vi "Dashboard Main.vi"() -> ()   [LabVIEW 2014]
uses:
  <vilib>/event_ctls.llb/eventvkey.ctl
  <vilib>/Utility/config.llb/NI_LVConfig.lvlib
  <vilib>/Utility/config.llb/Write Key (I32).vi
  <vilib>/Rock Robotics/WPI/Dashboard/WPI_DashboardLogging Global.vi
  <vilib>/Utility/config.llb/Write Key (String).vi
  <vilib>/Rock Robotics/Network Tables/SD Read Boolean.vi
  Support Files/Global Data!!!.vi
panel:
  in  "TCP":refnum<k5>
  in  "Rec Mode":enum32{"Stop", "Record", "Playback"}(radio)
  in  "Vision":u16(ring) items=["Camera Off", "USB Camera SW", "USB Camera HW", "IP Camera"]
  out "Camera IP":string
  out "Image Message":string="Timeout in Camera Communications"
  in  "Dashboard Tab":T1(tab)
  in  "Camera Settings":T2={"Frame Rate"=30, "Compression"=30, "Size"=1} {"Frame Rate" scale=1.0..30.0; "Size" items=["640x480", "320x240", "160x120"]}
  out "MotorChart R":cluster{"Numeric":dbl, "Numeric":dbl}(graph)
  out "MotorChart L":T3(graph)
  out "MotorSliders R":cluster{"MotorSlide1":dbl, "MotorSlide2":dbl} {"MotorSlide2" scale=-1.0..1.0 scale format="%#_2e"; "MotorSlide1" scale=-1.0..1.0 scale format="%#_2e"}
  out "MotorSliders L":T4 {"MotorSlide4 2" scale=0.0..14.0 scale format="%#_2e"; "MotorSlide2" scale=-1.0..1.0 scale format="%#_2e"; "MotorSlide1" scale=-1.0..1.0 scale format="%#_2e"}
  out "JS1 Z":dbl(slide) scale=-1.0..1.0 scale format="%#_2e"
  out "JS1 Graph":cluster{"X":dbl, "Y":dbl}[](graph)
  out "JS1 Buttons":T5
  out "JS2 Z":dbl(slide) scale=-1.0..1.0 scale format="%#_2e"
  out "JS2 Graph":cluster{"X":dbl, "Y":dbl}[](graph)
  out "JS2 Buttons":T5
  out "Mode":T6(ring)=enum."Auto Disabled"
  in  "DB Camera Config":bool
  out "fps":dbl format="%#.1g"
  out "Mbps":dbl format="%#.1g"
  out "Mbps 2":bool
  in  "DB/String 9":string
  in  "DB/String 8":string
  in  "DB/String 7":string
  in  "DB/String 6":string
  in  "DB/String 5":string
  in  "DB/String 4":string
  in  "DB/String 3":string
  in  "DB/String 2":string
  in  "DB/String 1":string
  in  "DB/String 0":string
  in  "DB/Slider 0":dbl(slide) scale=0.0..5.0
  in  "DB/Slider 1":dbl(slide) scale=0.0..5.0
  in  "DB/Slider 2":dbl(slide) scale=0.0..5.0
  in  "DB/Slider 3":dbl(slide) scale=0.0..5.0
  out "DB/LED 3":bool
  out "DB/LED 2":bool
  out "DB/LED 1":bool
  out "DB/LED 0":bool
  in  "DB/Button 3":bool
  in  "DB/Button 2":bool
  in  "DB/Button 1":bool
  in  "DB/Button 0":bool caption="New Name"
  out "BinTote":bool
  in  "Test Slider":dbl(slide) scale=0.0..100.0 scale format="%#_3g"
  in  "On/Off":bool caption="Solenoid"
  in  "Test Name":u16(ring) items=["Select the test to run...", "Example Test", "-------------------------------", "List of tests is built in robot code.", "Replace with your own automated tests."]
  in  "Test Tree":string(tree)
  in  "Motor":cluster{"Value":dbl, "Enable":bool} {"Value" scale=-1.0..1.0 scale format="%#_3g"}
  out "Progress":T7 {"Test Progress" scale=0.0..100.0}
  in  "Rev/Fwd":cluster{"Forward":bool, "Reverse":bool}
  in  "Test Ring":u16(ring) items=["Monochrome", "Color"]
  in  "Listbox":i32(listbox)
  out "Tree":string(tree)
  out "Camera Image":T8(plugin-control)
  out "Boolean":bool
  # "Left"
  # "Front"
  # "Right"
  # "Battery"
  # "This tab is a great place for autonomous settings and robot-specific values.\nPlace controls and indicators inside this tab and match name to\nDashboard Variables on robot. You can also delete this comment."
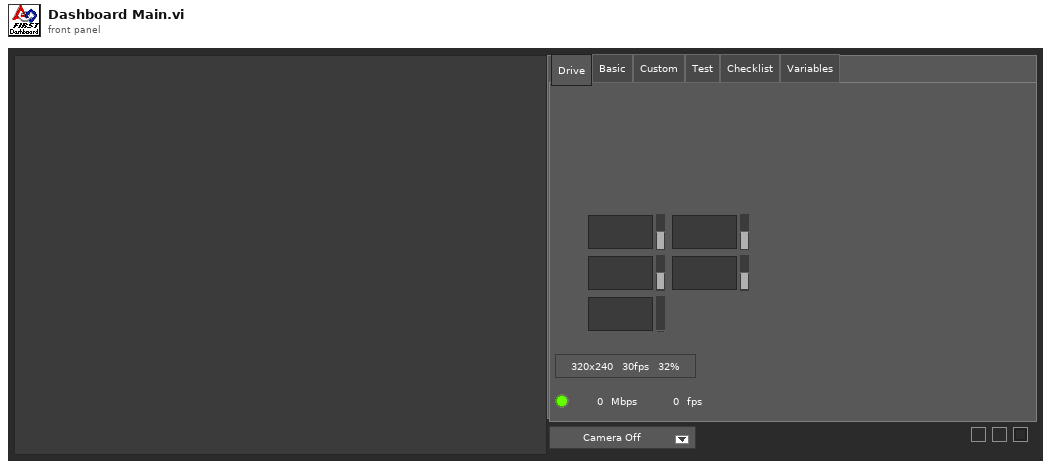
[diagram p1: front panel]
types:
  T1 = enum32{"Drive", "Basic", "Custom", "Test", "Checklist", "Variables"}
  T2 = cluster{"Frame Rate":i32, "Compression":i32, "Size":u16}
  T3 = cluster{"Numeric":dbl, "Numeric":dbl, "Battery V":dbl}
  T4 = cluster{"MotorSlide1":dbl, "MotorSlide2":dbl, "MotorSlide4 2":dbl}
  T5 = cluster{bool, bool, bool, bool, bool, bool, bool, bool, bool, bool, bool, bool}
  T6 = enum8{"Tele-Op Disabled", "Tele-Op Enabled", "Auto Disabled", "Auto Enabled", "Test Disabled", "Test Enabled", "Disconnected", "No Code", "E-Stop"}
  T7 = cluster{"Test Progress":u8, "Test Progress Text":string}
  T8 = typedef "IMAQ Image.ctl" = refnum<image>
  T9 = typedef "Image Type" = u32
  T10 = cluster{"Camera Image":refnum<vi>, "Dashboard Tab":refnum<vi>, "Boolean":refnum<vi>, "Vision":refnum<vi>, "Rec Mode":refnum<vi>, "Test Slider":refnum<vi>, "On/Off ":refnum<vi>, "Test Ring":refnum<vi>, "Rev/Fwd":refnum<vi>, "Test Name":refnum<vi>, "Motor":refnum<vi>, "Progress":refnum<vi>, "CheckList":refnum<vi>, "Tree":refnum<vi>, "Test Tree":refnum<vi>}
  T11 = cluster{"Error Strings":string, "Disable Counts":cluster{u16, u16}, "Rail Faults":cluster{u16, u16, u16}, "Robot IP":string, "DB Mode":u8, "Event Info":cluster{"Name":string, "Type":u8, "Number":u16, "Replay":u8}, "Camera Addr":string}
  T12 = cluster{"Storage":cluster{"Disk Free":u64, "RAM Block":u32, "RAM free":u32}, "CPU Utilization":cluster{"CPU % ISR":sgl, "CPU % Time Crit":sgl, "CPU % Timed Str":sgl, "CPU % High":sgl, "CPU % Above":sgl, "CPU % Normal":sgl, "CPU % Low":sgl}, "CAN":cluster{"% Bus Utilization":sgl, "Bus Off Cnt":u32, "TX_FIFO Full Cnt":u32, "Receive Error Cnt":u8, "Transmit Error Cnt":u8}, "HID":cluster{"HID Outputs":u32, "Rumble Low":u16, "Rumble High":u16}[]}
  T13 = cluster{"Status bits":cluster{"Test Mode":bool, "Autonomous":bool, "Enabled":bool, "Code Start":bool, "Brownout":bool, "Reserved 2":bool, "Reserved 3":bool, "E-Stop":bool}, "Code Trace":cluster{"Disabled":bool, "TeleOp":bool, "Auto":bool, "Test":bool}, "Controller Type":enum16{"unknown", "cRIO", "roboRio"}, "Code?":enum16{"unknown", "noCode", "code"}, "Battery V":dbl}
  T14 = cluster{"Control Bits":cluster{"TestMode":bool, "Autonomous":bool, "Enabled":bool, "FMS Present":bool, bool, bool, bool, "E-Stop":bool}, "Team Station ":u8, "Countdown":sgl, "Joystick Values":cluster{"Axes":dbl[], "Buttons":bool[], "POVs":i16[]}[]}
  T15 = cluster{"Axes":dbl[], "Buttons":bool[], "POVs":i16[]}[]
  T16 = cluster{"Axes":dbl[], "Buttons":bool[], "POVs":i16[]}
  T17 = cluster{"Buttons[0]":bool, "Buttons[1]":bool, "Buttons[2]":bool, "Buttons[3]":bool, "Buttons[4]":bool, "Buttons[5]":bool, "Buttons[6]":bool, "Buttons[7]":bool, "Buttons[8]":bool, "Buttons[9]":bool, "Buttons[10]":bool, "Buttons[11]":bool}
  T18 = typedef "NI_LVConfig.lvlib/Config Data RefNum.ctl" = refnum<k1>
  T19 = cluster{"Operation":enum16{"Update", "Clear"}, "Color Box":u32}[]
  T20 = typedef "eventvkey.ctl" = enum16{"ASCII", "Enter", "Return", "Shift", "Ctrl", "Alt", "Cmd", "Opt", "Caps", "NumLock", "Clear", "Break", "Up", "Down", "Left", "Right", "Insert", "Delete", "Home", "End", "PageUp", "PageDown", "Escape", "Help", "Pause", "ScrollLock", "F1", "F2", "F3", "F4", "F5", "F6", "F7", "F8", "F9", "F10", "F11", "F12", "F13", "F14", "F15", "F16", "F17", "F18", "F19", "F20", "F21", "F22", "F23", "F24", "Play", "VolumeUp", "VolumeDown", "Mute", "Two Byte Char"}
  T21 = cluster{"Image Size":bool, "Image Type":bool, "Pixel Value":bool, "ROI Information":bool, "Zoom Factor":bool}
  T22 = enum8{"Enabled", "Disabled", "Disabled and Grayed Out"}
  T23 = cluster{"Operation":enum16{"Update", "Clear"}, "Color Box":u32}
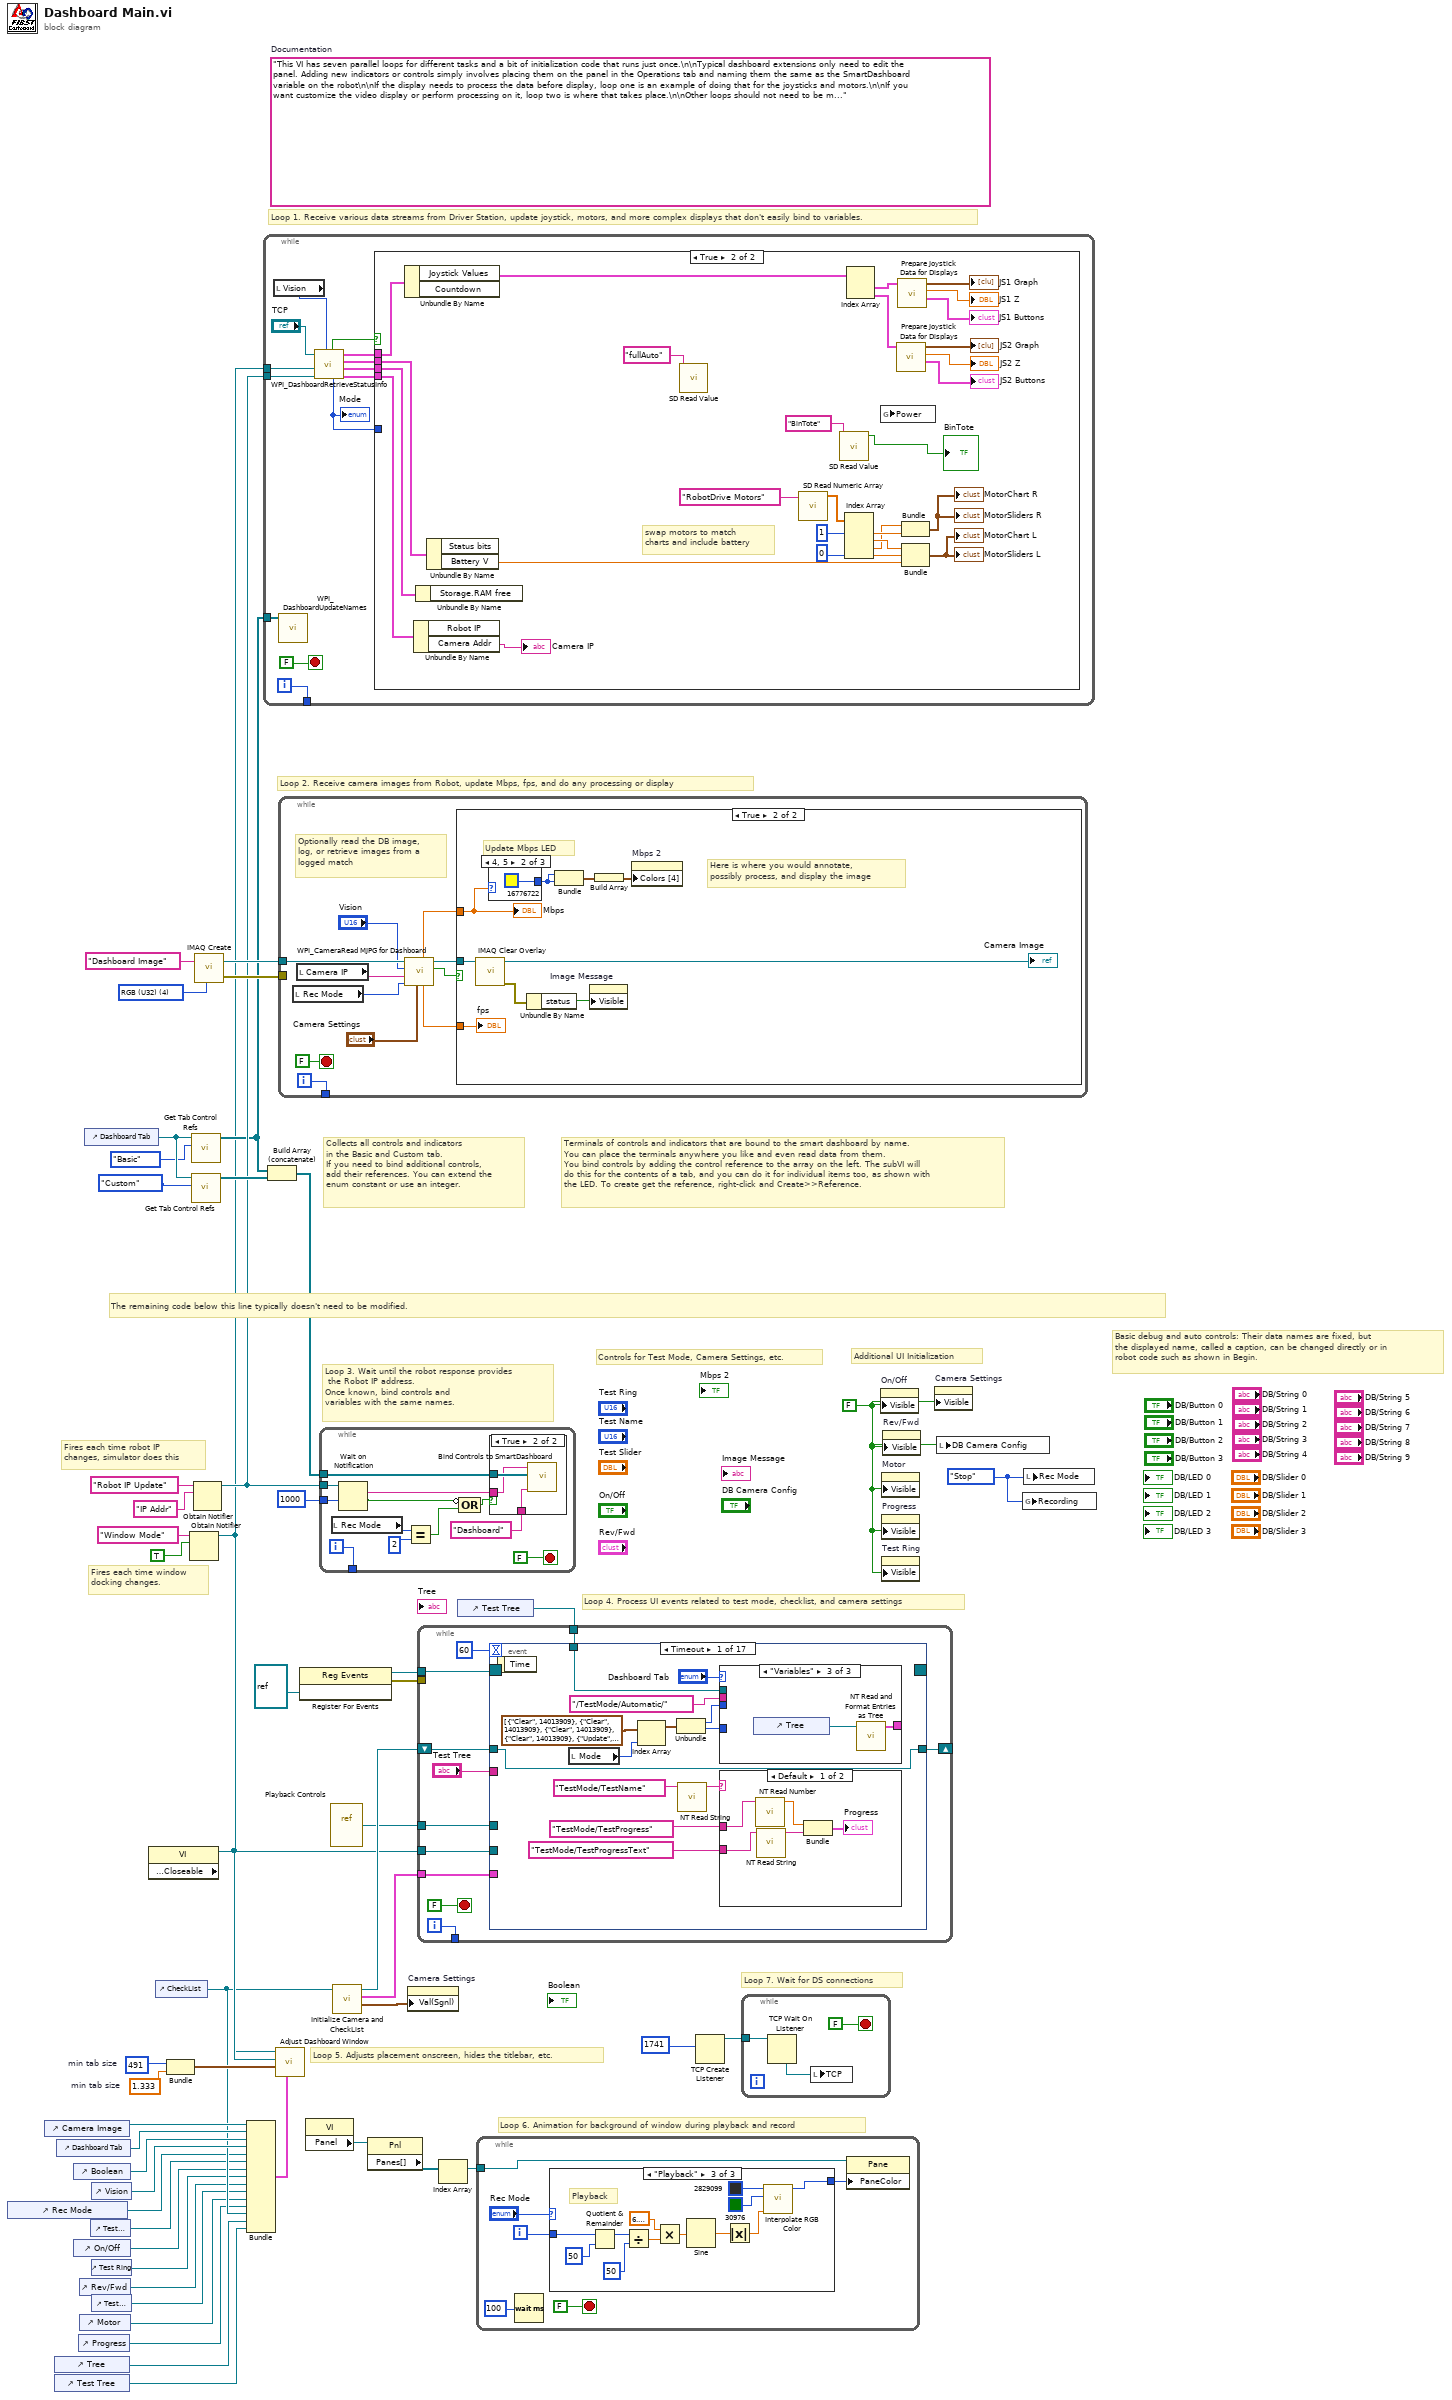
[diagram p0: block diagram]
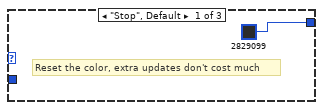
[diagram p3: hidden frame]
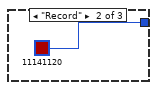
[diagram p4: hidden frame]
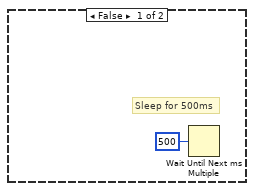
[diagram p6: hidden frame]
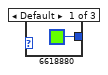
[diagram p7: hidden frame]
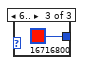
[diagram p8: hidden frame]
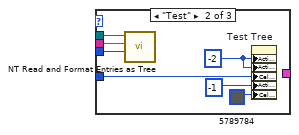
[diagram p10: hidden frame]
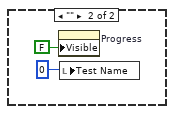
[diagram p11: hidden frame]
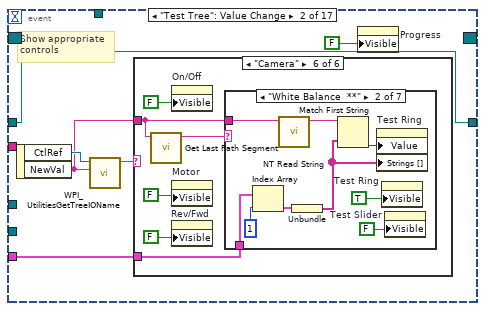
[diagram p12: hidden frame]
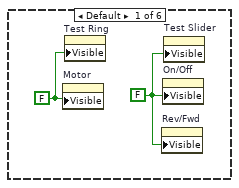
[diagram p13: hidden frame]
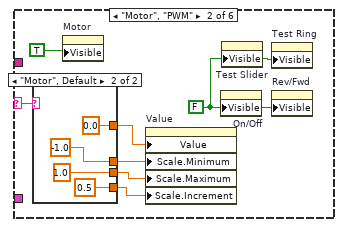
[diagram p14: hidden frame]
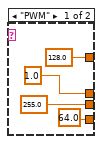
[diagram p15: hidden frame]
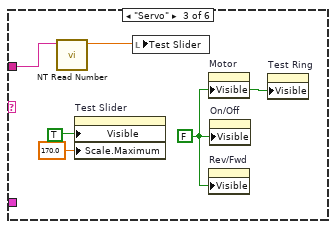
[diagram p16: hidden frame]
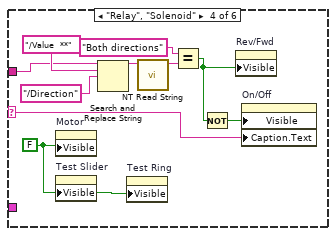
[diagram p17: hidden frame]
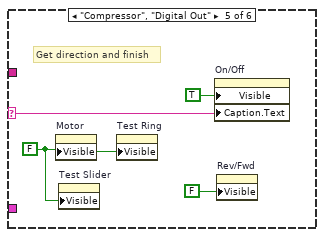
[diagram p18: hidden frame]
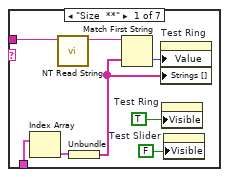
[diagram p19: hidden frame]
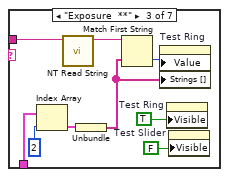
[diagram p20: hidden frame]
diagram:
  w24 = 491  # min tab size
  w23 = 1.333  # min tab size
  w32 = enum32{"Stop", "Record", "Playback"}."Stop" ("Rec Mode")
  w6 = FALSE ("Visible")
  (unwired) "This VI has seven parallel loops for different tasks and a bit of initialization code that runs just once.\n\nTypical dashboard extensions only need to edit the panel. Adding new indicators or controls simply involves placing them on the panel in the Operations tab and naming them the same as the SmartDashboard variable on the robot\n\nIf the display needs to process the data before display, loop one is an example of doing that for the joysticks and motors.\n\nIf you want customize the video display or perform processing on it, loop two is where that takes place.\n\nOther loops should not need to be modified. They are pretty standard, and document the task they perform."  # Documentation
  w52 = T9 4 items=["Grayscale (U8)", "Grayscale (I16)", "Grayscale (SGL)", "Complex (CSG)", "RGB (U32)", "HSL (U32)", "RGB (U64)"] ("Image Type")
  # "Loop 7. Wait for DS connections"
  # "Basic debug and auto controls: Their data names are fixed, but\nthe displayed name, called a caption, can be changed directly or in\nrobot code such as shown in Begin."
  # "Controls for Test Mode, Camera Settings, etc."
  # "Additional UI Initialization"
  # "Loop 6. Animation for background of window during playback and record"
  # "Fires each time robot IP\nchanges, simulator does this"
  # "Fires each time window\ndocking changes."
  # "Collects all controls and indicators\nin the Basic and Custom tab.\nIf you need to bind additional controls,\nadd their references. You can extend the\nenum constant or use an integer."
  # "The remaining code below this line typically doesn't need to be modified."
  # "Loop 4. Process UI events related to test mode, checklist, and camera settings"
  # "Terminals of controls and indicators that are bound to the smart dashboard by name.\nYou can place the terminals anywhere you like and even read data from them.\nYou bind controls by adding the control reference to the array on the left. The subVI will\ndo this for the contents of a tab, and you can do it for individual items too, as shown with\nthe LED. To create get the reference, right-click and Create>>Reference."
  # "Loop 3. Wait until the robot response provides\n the Robot IP address.\nOnce known, bind controls and\nvariables with the same names."
  # "Loop 5. Adjusts placement onscreen, hides the titlebar, etc."
  # "Loop 1. Receive various data streams from Driver Station, update joystick, motors, and more complex displays that don't easily bind to variables."
  # "Loop 2. Receive camera images from Robot, update Mbps, fps, and do any processing or display"
  n1 = control-ref of="Rec Mode"() -> (w12:refnum<vi>)
  n2 = control-ref of="Camera Image"() -> (w27:refnum<vi>)
  n3 = control-ref of="Tree"() -> (w16:refnum<vi>)
  n4 = control-ref of="Test Tree"() -> (w15:refnum<vi>)
  n5 = control-ref of="Dashboard Tab"() -> (w26:refnum<vi>)
  n6 = control-ref of="Boolean"() -> (w21:refnum<vi>)
  n7 = control-ref of="On/Off"() -> (w10:refnum<vi>)
  n8 = control-ref of="Progress"() -> (w7:refnum<vi>)
  n9 = control-ref of="Rev/Fwd"() -> (w8:refnum<vi>)
  n10 = control-ref of="Motor"() -> (w13:refnum<vi>)
  n11 = control-ref of="Dashboard Tab"() -> (w30:refnum<vi>)
  n12 = control-ref of="Test Slider"() -> (w11:refnum<vi>)
  n13 = control-ref of="Vision"() -> (w25:refnum<vi>)
  n14 = control-ref of="Test Ring"() -> (w9:refnum<vi>)
  n15 = control-ref of="Test Name"() -> (w14:refnum<vi>)
  n16 = property class="VI" props=["Front Panel.Closeable"]() -> (reference out=w31:refnum<vi>)  [unwired: 2 in, 2 out]
  n17 = control-ref of="CheckList"() -> (w17:refnum<vi>)
  n18 = Bundle("min tab size"=w24, "min tab size"=w23) -> (w22:cluster{"min tab size":i32, "min tab size":dbl})  [unwired: 1 in]
  n19 = Obtain Notifier(name (unnamed)="Window Mode", notification data type=TRUE) -> (notifier out=w3:refnum<notifier>)  [unwired: 2 in, 2 out]
  n20 = call <vilib>:"Get Tab Control Refs.vi"("Page Index"=T1."Basic" ("Dashboard Tab"), "TabControl in"=w30) -> ("ControlsOnPage"=w4:refnum<vi>[])  [unwired: 9 in]
  n21 = call <vilib>:"Get Tab Control Refs.vi"("Page Index"=T1."Custom" ("Dashboard Tab"), "TabControl in"=w30) -> ("ControlsOnPage"=w29:refnum<vi>[])  [unwired: 9 in]
  n22 = Obtain Notifier(name (unnamed)="Robot IP Update", notification data type="IP Addr" ("name (unnamed)")) -> (notifier out=w5:refnum<notifier>)  [unwired: 2 in, 2 out]
  n23 = call "IMAQ Create"("Image Name"="Dashboard Image", "Image Type"=w52) -> ("New Image"=w50:T8, "error out"=w49:errorcluster)  [unwired: 2 in, 1 out]
  n24 = Bundle("Camera Image"=w27, "Dashboard Tab"=w26, "Boolean"=w21, "Vision"=w25, "Rec Mode"=w12, "Test Slider"=w11, "On/Off"=w10, "Test Ring"=w9, "Rev/Fwd"=w8, "Test Name"=w14, "Motor"=w13, "Progress"=w7, "CheckList"=w17, "Tree"=w16, "Test Tree"=w15) -> (w18:T10)  [unwired: 1 in]
  n25 = while {
    tunnel: [w64] -> _
    tunnel: w5 -> [w58]
    tunnel: w4 -> [w57]
    tunnel: w3 -> [w53]
    i -> [w64]
    stop <- FALSE stop-if-true
    n26 = local read "Vision"() -> (w55:u16)
    n27 = call <vilib>:"WPI_DashboardUpdateNames.vi"("Controls on Tab"=w57) -> ()  [unwired: 11 in]
    n28 = call <vilib>:"WPI_DashboardRetrieveStatusInfo.vi"("Vision"=w55, "Binding Refnum"=w58, "Window Mode Notifier"=w53, "TCP Cnx"="TCP") -> ("Power and Errors"=w59:T11, "Robot Metrics"=w62:T12, "Status Info"=w63:T13, "Control Info"=w60:T14, "Robot Mode"=w56:T6, "Process?"=w61:bool)  [unwired: 2 in]
    "Mode" <- w56
    n29 = case shown="True" w61 {
      tunnel: w63 -> [_ w93]
      tunnel: w62 -> [_ w92]
      tunnel: w60 -> [_ w91]
      tunnel: w59 -> [_ w90]
      tunnel: w56 -> [_ _]
      frame False {
      }
      frame True {
        # "swap motors to match\ncharts and include battery"
        n30 = Unbundle By Name(w91) -> ("Joystick Values"=w78:T15)  [unwired: 1 out]
        n31 = Unbundle By Name(w90) -> ("Camera Addr"=→"Camera IP":string)  [unwired: 1 out]
        n32 = Unbundle By Name(w92) -> ()  [unwired: 1 out]
        n33 = Unbundle By Name(w93) -> ("Battery V"=w79:dbl)  [unwired: 1 out]
        n34 = call-poly <vilib>:"SD Read Value.vi"("Name"="fullAuto") -> ()  [unwired: 8 in, 3 out]
        n35 = call <vilib>:"SD Read Numeric Array.vi"("Name"="RobotDrive Motors") -> ("Numeric Array"=w81:dbl[])  [unwired: 8 in, 2 out]
        n36 = call-poly <vilib>:"SD Read Value.vi"("Name"="BinTote") -> ("Boolean"=→"BinTote":bool)  [unwired: 8 in, 2 out]
        n37 = Index Array(array=w81, index #1=1, index #4=0) -> (element #1=w85:dbl, element #2=w86:dbl, element #3=w84:dbl, element #4=w89:dbl)  [unwired: 2 in]
        n38 = Index Array(array=w78) -> (element #1=w77:T16, element #2=w72:T16)  [unwired: 2 in]
        n39 = global read "Global Data!!!.vi" "Power"() -> ()  [unwired: 1 in]
        n40 = call "Prepare Joystick Data for Displays.vi"("Joystick Values"=w72) -> ("Buttons"=→"JS2 Buttons":T17, "Z Axis"=→"JS2 Z":dbl, "Cartesian Data"=→"JS2 Graph":cluster{"X axis":dbl, "X axis":dbl}[])  [unwired: 8 in]
        n41 = call "Prepare Joystick Data for Displays.vi"("Joystick Values"=w77) -> ("Buttons"=→"JS1 Buttons":T17, "Z Axis"=→"JS1 Z":dbl, "Cartesian Data"=→"JS1 Graph":cluster{"X axis":dbl, "X axis":dbl}[])  [unwired: 8 in]
        n42 = Bundle("Numeric"=w84, "Numeric"=w85) -> (→"MotorChart R" →"MotorSliders R":cluster{"Numeric":dbl, "Numeric":dbl})  [unwired: 1 in]
        n43 = Bundle("Numeric"=w86, "Numeric"=w89, "Battery V"=w79) -> (→"MotorChart L" →"MotorSliders L":T3)  [unwired: 1 in]
      }
    }
  }
  n44 = Build Array (concatenate)(w4, w29) -> (w28:refnum<vi>[])
  n45 = call "Adjust Dashboard Window.vi"("Sizing Refnums"=w18, "Size Constraints"=w22, "VI"=w31, "Notifier in"=w3) -> ()  [unwired: 8 in]
  n46 = while {
    tunnel: w50 -> [w102]
    tunnel: w49 -> [_]
    tunnel: [w103] -> _
    i -> [w103]
    stop <- FALSE stop-if-true
    # "Optionally read the DB image,\nlog, or retrieve images from a\nlogged match"
    n47 = local read "Rec Mode"() -> (w96:enum32{"Stop", "Record", "Playback"})
    n48 = local read "Camera IP"() -> (w94:string)
    n49 = call <vilib>:"WPI_CameraRead MJPG for Dashboard.vi"("Camera Settings"="Camera Settings", "Rec Mode"=w96, "Camera IP"=w94, "Camera Mode"="Vision", "Refnum in"=w102) -> ("Active"=w100:bool, "Refnum out"=w101:T8, "FPS"=w99:dbl, "Bandwidth (Mbps)"=w98:dbl)  [unwired: 3 in]
    n50 = case shown="True" w100 {
      tunnel: w101 -> [_ w109]
      tunnel: w98 -> [_ w108]
      tunnel: w99 -> [_ w106]
      frame False {
        # "Sleep for 500ms"
        n51 = Wait Until Next ms Multiple(millisecond multiple=u32 500) -> ()  [unwired: 1 out]
      }
      frame True {
        # "Here is where you would annotate,\npossibly process, and display the image"
        # "Update Mbps LED"
        n52 = call "IMAQ Clear Overlay"("Image"=w109) -> ("error out"=w113:errorcluster, "Image Out"=→"Camera Image":T8)  [unwired: 2 in, 7 out]
        n53 = case shown="4, 5" w108 {
          tunnel: [u32 6618880 ("Color Box") u32 16776722 ("Color Box") u32 16716800 ("Color Box")] -> w110
          frame Default {
          }
          frame 4, 5 {
          }
          frame 6.. {
          }
        }
        n54 = Unbundle By Name(w113) -> ("status"=w114:bool)
        n55 = Bundle("Color Box"=w110, "Color Box"=w110) -> (w112:cluster{"Color Box":u32, "Color Box":u32})  [unwired: 1 out]
        n56 = property on="Image Message" class="Str"("Visible"=w114) -> ()  [unwired: 2 in, 2 out]
        n57 = Build Array(w112) -> (w111:cluster{"Color Box":u32, "Color Box":u32}[])
        n58 = property on="Mbps 2" class="Bool (strict)"("Colors [4]"=w111) -> ()  [unwired: 2 in, 2 out]
        "Mbps" <- w108
        "fps" <- w106
      }
    }
  }
  n59 = register-events(refnum<vi> refnum) -> (reference out=w36:refnum<event-registration>, error out=w35:errorcluster)  [unwired: 2 in]
  n60 = property class="VI"() -> ("Panel"=w39:refnum<vi>)  [unwired: 2 in, 2 out]
  n61 = while {
    tunnel: w28 -> [w129]
    tunnel: w5 -> [w127]
    tunnel: [w125] -> _
    tunnel: u32 1000 ("milliseconds to wait") -> [w124]
    i -> [w125]
    stop <- FALSE stop-if-true
    n62 = local read "Rec Mode"() -> (w120:enum32{"Stop", "Record", "Playback"})
    n63 = Wait on Notification(notifier=w127, timeout in ms (-1)=w124) -> (notification=w126:string, timed out?=w122:bool)  [unwired: 2 in, 2 out]
    n64 = Equal?(x=w120, y=u16 2 ("Rec Mode")) -> (x = y?=w121:bool)
    n65 = Compound Arithmetic op=OR(invert w122, w121) -> (w123:bool)
    n66 = case shown="True" w123 {
      tunnel: w129 -> [_ w132]
      tunnel: w126 -> [_ w131]
      tunnel: "Dashboard" -> [_ w130]
      frame False {
      }
      frame True {
        n67 = call <vilib>:"Bind Controls to SmartDashboard.vi"("Client Name"=w130, "Bound Control Refs"=w132, "Server IP Address"=w131) -> ()  [unwired: 9 in]
      }
    }
  }
  n68 = vi-ref "Playback Controls.vi"() -> (w37:refnum<vi>)
  n69 = call "Initialize Camera and CheckList.vi"("ListBox in"=w17) -> ("Cluster"=w43:cluster{"value":i32, "value":i32, "index":i32}, "Array"=w44:cluster{string[]}[], "File Refnum"=w42:T18)  [unwired: 8 in]
  n70 = property class="Pnl"(reference=w39) -> ("Panes[]"=w40:refnum<vi>[])  [unwired: 1 in, 2 out]
  n71 = property on="Camera Settings" class="Clust (strict)"("Val(Sgnl)"=w43) -> ()  [unwired: 2 in, 2 out]
  n72 = Index Array(array=w40) -> (element=w38:refnum<vi>)  [unwired: 1 in]
  n73 = control-ref of="Test Tree"() -> (w41:refnum<vi>)
  n74 = while {
    tunnel: w44 -> [w140]
    shift-right: [w139] -> _
    shift-left: w42 -> [w138]
    tunnel: [w137] -> _
    tunnel: w41 -> [w136]
    tunnel: w37 -> [w135]
    tunnel: w36 -> [w134]
    tunnel: w35 -> [_]
    tunnel: w31 -> [w133]
    i -> [w137]
    stop <- FALSE stop-if-true
    n75 = event shown="[0] Timeout" {
      selector: w134 -> [_ _ _ _ _ _ _ _ _ _ _ _ _ _ _ _ _]
      dyn-events: [_ _ _ _ _ _ _ _ _ _ _ _ _ w378 _ _ _] -> _
      timeout: u32 60 ("milliseconds to wait") -> [_ _ _ _ _ _ _ _ _ _ _ _ _ _ _ _ _]
      tunnel: w136 -> [w152 _ _ _ _ _ _ _ _ _ _ _ _ _ _ _ _]
      tunnel: "Test Tree" -> [_ _ _ _ _ _ _ _ w347 w355 w357 w361 w369 _ _ _ _]
      tunnel: w140 -> [_ w174 _ _ _ _ w311 w341 _ _ _ _ _ _ _ _ _]
      tunnel: [w148 w173 w272 w277 w285 w297 w310 w334 w346 w353 w356 w360 w368 w380 w394 w395 w405] -> w139
      tunnel: w138 -> [w148 w173 w272 w277 w285 w297 w309 w334 w346 w353 w356 w360 w368 w380 w394 w395 w405]
      tunnel: w135 -> [_ _ _ _ _ _ _ _ _ _ _ _ _ w381 _ w398 _]
      tunnel: w133 -> [_ _ _ _ _ _ _ _ _ _ _ _ _ w376 _ _ _]
      event Timeout {
        n76 = event-data() -> ()  [unwired: 1 in, 1 out]
        n77 = local read "Mode"() -> (w151:T6)
        n78 = Index Array(array=T19 [{"Operation"=enum."Clear", "Color Box"=14013909}, {"Operation"=enum."Clear", "Color Box"=14013909}, {"Operation"=enum."Clear", "Color Box"=14013909}, {"Operation"=enum."Clear", "Color Box"=14013909}, {"Operation"=enum."Update", "Color Box"=14013909}, {"Operation"=enum."Update", "Color Box"=16777215}, {"Operation"=enum."Clear", "Color Box"=14013909}, {"Operation"=enum."Clear", "Color Box"=14013909}, {"Operation"=enum."Clear", "Color Box"=14013909}], index=w151) -> (element=w146:T23)
        n79 = Unbundle(w146) -> ("Operation"=w145:enum16{"Update", "Clear"}, "Color Box"=w144:u32)
        n80 = call <vilib>:"NT Read String.vi"("Name"="TestMode/TestName") -> ("String"=w155:string)  [unwired: 9 in, 1 out]
        n81 = case shown="\"Variables\"" "Dashboard Tab" {
          tunnel: w152 -> [_ w163 _]
          tunnel: "/TestMode/Automatic/" ("Name Pattern") -> [_ w162 _]
          tunnel: w145 -> [_ w161 _]
          tunnel: [_ _ w165] -> _
          tunnel: w144 -> [_ w157 _]
          frame "Custom", Default {
          }
          frame "Test" {
            w160 = -2 ("Active Item:Row Number")
            n82 = call <vilib>:"NT Read and Format Entries as Tree.vi"("Operation"=w161, "Name Pattern"=w162, "Tree Refnum"=w163) -> ()  [unwired: 7 in, 2 out]
            n83 = property on="Test Tree" class="Tree (strict)"("Active Item Row Number"=w160, "ActiveColNum"=w160, "CellBG"=w157, "Active Item Row Number"=-1 ("Active Item:Row Number"), "CellBG"=u32 5789784 ("Color Box")) -> ()  [unwired: 2 in, 2 out]
          }
          frame "Variables" {
            n84 = control-ref of="Tree"() -> (w164:refnum<vi>)
            n85 = call <vilib>:"NT Read and Format Entries as Tree.vi"("Tree Refnum"=w164) -> ("Formatted Strings"=w165:cluster{"Name":string, "Value":string}[])  [unwired: 9 in, 1 out]
          }
        }
        n86 = case shown="Default" w155 {
          tunnel: "TestMode/TestProgress" ("Name") -> [w167 _]
          tunnel: "TestMode/TestProgressText" ("Name") -> [w166 _]
          frame Default {
            n87 = call <vilib>:"NT Read Number.vi"("Name"=w167) -> ("Numeric"=w168:dbl)  [unwired: 9 in, 1 out]
            n88 = call <vilib>:"NT Read String.vi"("Name"=w166) -> ("String"=w169:string)  [unwired: 9 in, 1 out]
            n89 = Bundle("Numeric"=w168, "String"=w169) -> (→"Progress":cluster{"Numeric":dbl, "String":string})  [unwired: 1 in]
          }
          frame "" {
            n90 = property on="Progress" class="Clust (strict)"("Visible"=FALSE) -> ()  [unwired: 2 in, 2 out]
            n91 = local write "Test Name"(u16 0) -> ()
          }
        }
      }
      event "Test Tree": Value Change {
        # "Show appropriate\ncontrols"
        n92 = event-data() -> ("CtlRef"=w177:refnum<vi>, "NewVal"=w175:string)  [unwired: 1 in]
        n93 = call <vilib>:"WPI_UtilitiesGetTreeIOName.vi"("NewVal"=w175, "TreeControl in"=w177) -> ("I/O Name"=w178:string)  [unwired: 9 in]
        n94 = case shown="\"Camera\"" w178 {
          selector: w178 -> [_ w185 _ w203 w212 _]
          tunnel: w175 -> [_ _ w200 w202 _ w219]
          tunnel: w174 -> [_ _ _ _ _ w218]
          frame Default {
            w180 = FALSE ("Visible")
            w179 = FALSE ("Visible")
            n95 = property on="Motor" class="Clust (strict)"("Visible"=w179) -> ()  [unwired: 2 in, 2 out]
            n96 = property on="Test Ring" class="Ring (strict)"("Visible"=w179) -> ()  [unwired: 2 in, 2 out]
            n97 = property on="Rev/Fwd" class="Clust (strict)"("Visible"=w180) -> ()  [unwired: 2 in, 2 out]
            n98 = property on="On/Off" class="Bool (strict)"("Visible"=w180) -> ()  [unwired: 2 in, 2 out]
            n99 = property on="Test Slider" class="Slide (strict)"("Visible"=w180) -> ()  [unwired: 2 in, 2 out]
          }
          frame "Motor", "PWM" {
            w186 = FALSE ("Visible")
            n100 = case shown="\"Motor\", Default" w185 {
              tunnel: [1.0 ("Value") -1.0 ("Value")] -> w184
              tunnel: [255.0 ("Value") 1.0 ("Value")] -> w183
              tunnel: [128.0 ("Value") 0.0 ("Value")] -> w182
              tunnel: [64.0 ("Value") 0.5 ("Value")] -> w181
              frame "PWM" {
              }
              frame "Motor", Default {
              }
            }
            n101 = property on="Motor" class="Clust (strict)"("Visible"=TRUE) -> ()  [unwired: 2 in, 2 out]
            n102 = property on="Value" class="Slide (strict)"("Value"=w182, "Scale.Minimum"=w184, "Scale.Maximum"=w183, "Scale.Increment"=w181) -> ()  [unwired: 2 in, 2 out]
            n103 = property on="On/Off" class="Bool (strict)"("Visible"=w186) -> ()  [unwired: 2 in, 2 out]
            n104 = property on="Test Slider" class="Slide (strict)"("Visible"=w186) -> ()  [unwired: 2 in, 2 out]
            n105 = property on="Test Ring" class="Ring (strict)"("Visible"=w186) -> ()  [unwired: 2 in, 2 out]
            n106 = property on="Rev/Fwd" class="Clust (strict)"("Visible"=w186) -> ()  [unwired: 2 in, 2 out]
          }
          frame "Servo" {
            w198 = FALSE ("Visible")
            n107 = call <vilib>:"NT Read Number.vi"("Name"=w200) -> ("Numeric"=w199:dbl)  [unwired: 9 in, 1 out]
            n108 = property on="Test Slider" class="Slide (strict)"("Visible"=TRUE, "Scale.Maximum"=170.0 ("Scale.Range:Maximum")) -> ()  [unwired: 2 in, 2 out]
            n109 = local write "Test Slider"(w199) -> ()
            n110 = property on="Motor" class="Clust (strict)"("Visible"=w198) -> ()  [unwired: 2 in, 2 out]
            n111 = property on="Rev/Fwd" class="Clust (strict)"("Visible"=w198) -> ()  [unwired: 2 in, 2 out]
            n112 = property on="On/Off" class="Bool (strict)"("Visible"=w198) -> ()  [unwired: 2 in, 2 out]
            n113 = property on="Test Ring" class="Ring (strict)"("Visible"=w198) -> ()  [unwired: 2 in, 2 out]
          }
          frame "Relay", "Solenoid" {
            w201 = FALSE ("Visible")
            n114 = property on="Motor" class="Clust (strict)"("Visible"=w201) -> ()  [unwired: 2 in, 2 out]
            n115 = property on="Test Slider" class="Slide (strict)"("Visible"=w201) -> ()  [unwired: 2 in, 2 out]
            n116 = Search and Replace String(input string=w202, search string="/Value  **", replace string="/Direction") -> (result string=w208:string)  [unwired: 5 in, 3 out]
            n117 = property on="Test Ring" class="Ring (strict)"("Visible"=w201) -> ()  [unwired: 2 in, 2 out]
            n118 = call <vilib>:"NT Read String.vi"("Name"=w208) -> ("String"=w206:string)  [unwired: 9 in, 1 out]
            n119 = Equal?(x="Both directions", y=w206) -> (x = y?=w204:bool)
            n120 = Not(x=w204) -> (.not. x?=w205:bool)
            n121 = property on="Rev/Fwd" class="Clust (strict)"("Visible"=w204) -> ()  [unwired: 2 in, 2 out]
            n122 = property on="On/Off" class="Bool (strict)"("Visible"=w205, "Caption.Text"=w203) -> ()  [unwired: 2 in, 2 out]
          }
          frame "Compressor", "Digital Out" {
            w211 = FALSE ("Visible")
            # "Get direction and finish"
            n123 = property on="Motor" class="Clust (strict)"("Visible"=w211) -> ()  [unwired: 2 in, 2 out]
            n124 = property on="Test Slider" class="Slide (strict)"("Visible"=w211) -> ()  [unwired: 2 in, 2 out]
            n125 = property on="Test Ring" class="Ring (strict)"("Visible"=w211) -> ()  [unwired: 2 in, 2 out]
            n126 = property on="On/Off" class="Bool (strict)"("Visible"=TRUE, "Caption.Text"=w212) -> ()  [unwired: 2 in, 2 out]
            n127 = property on="Rev/Fwd" class="Clust (strict)"("Visible"=FALSE) -> ()  [unwired: 2 in, 2 out]
          }
          frame "Camera" {
            n128 = call <vilib>:"Get Last Path Segment.vi"("String in"=w219) -> ("String out"=w220:string)  [unwired: 10 in]
            n129 = property on="On/Off" class="Bool (strict)"("Visible"=FALSE) -> ()  [unwired: 2 in, 2 out]
            n130 = property on="Motor" class="Clust (strict)"("Visible"=FALSE) -> ()  [unwired: 2 in, 2 out]
            n131 = property on="Rev/Fwd" class="Clust (strict)"("Visible"=FALSE) -> ()  [unwired: 2 in, 2 out]
            n132 = case shown="\"White Balance  **\"" w220 {
              tunnel: w219 -> [w226 w235 w244 w253 w262 _ w268]
              tunnel: w218 -> [w224 w232 w241 w250 w259 _ _]
              frame "Size  **" {
                n133 = Index Array(array=w224) -> (element=w223:cluster{string[]})  [unwired: 1 in]
                n134 = call <vilib>:"NT Read String.vi"("Name"=w226) -> ("String"=w225:string)  [unwired: 9 in, 1 out]
                n135 = Unbundle(w223) -> (w221:string[])
                n136 = Match First String(2:w221, 3:w225) -> (0:w222:i32)  [unwired: 1 out]
                n137 = property on="Test Ring" class="Ring (strict)"("Value"=w222, "Strings []"=w221) -> ()  [unwired: 2 in, 2 out]
                n138 = property on="Test Ring" class="Ring (strict)"("Visible"=TRUE) -> ()  [unwired: 2 in, 2 out]
                n139 = property on="Test Slider" class="Slide (strict)"("Visible"=FALSE) -> ()  [unwired: 2 in, 2 out]
              }
              frame "White Balance  **" {
                n140 = Index Array(array=w232, index=1) -> (element=w233:cluster{string[]})
                n141 = call <vilib>:"NT Read String.vi"("Name"=w235) -> ("String"=w234:string)  [unwired: 9 in, 1 out]
                n142 = Unbundle(w233) -> (w230:string[])
                n143 = Match First String(2:w230, 3:w234) -> (0:w229:i32)  [unwired: 1 out]
                n144 = property on="Test Ring" class="Ring (strict)"("Value"=w229, "Strings []"=w230) -> ()  [unwired: 2 in, 2 out]
                n145 = property on="Test Ring" class="Ring (strict)"("Visible"=TRUE) -> ()  [unwired: 2 in, 2 out]
                n146 = property on="Test Slider" class="Slide (strict)"("Visible"=FALSE) -> ()  [unwired: 2 in, 2 out]
              }
              frame "Exposure  **" {
                n147 = Index Array(array=w241, index=2) -> (element=w242:cluster{string[]})
                n148 = call <vilib>:"NT Read String.vi"("Name"=w244) -> ("String"=w243:string)  [unwired: 9 in, 1 out]
                n149 = Unbundle(w242) -> (w238:string[])
                n150 = Match First String(2:w238, 3:w243) -> (0:w239:i32)  [unwired: 1 out]
                n151 = property on="Test Ring" class="Ring (strict)"("Value"=w239, "Strings []"=w238) -> ()  [unwired: 2 in, 2 out]
                n152 = property on="Test Ring" class="Ring (strict)"("Visible"=TRUE) -> ()  [unwired: 2 in, 2 out]
                n153 = property on="Test Slider" class="Slide (strict)"("Visible"=FALSE) -> ()  [unwired: 2 in, 2 out]
              }
              frame "Exposure Priority  **" {
                n154 = Index Array(array=w250, index=3) -> (element=w251:cluster{string[]})
                n155 = call <vilib>:"NT Read String.vi"("Name"=w253) -> ("String"=w252:string)  [unwired: 9 in, 1 out]
                n156 = Unbundle(w251) -> (w247:string[])
                n157 = Match First String(2:w247, 3:w252) -> (0:w248:i32)  [unwired: 1 out]
                n158 = property on="Test Ring" class="Ring (strict)"("Value"=w248, "Strings []"=w247) -> ()  [unwired: 2 in, 2 out]
                n159 = property on="Test Ring" class="Ring (strict)"("Visible"=TRUE) -> ()  [unwired: 2 in, 2 out]
                n160 = property on="Test Slider" class="Slide (strict)"("Visible"=FALSE) -> ()  [unwired: 2 in, 2 out]
              }
              frame "Color Enable  **" {
                n161 = Index Array(array=w259, index=4) -> (element=w260:cluster{string[]})
                n162 = call <vilib>:"NT Read String.vi"("Name"=w262) -> ("String"=w261:string)  [unwired: 9 in, 1 out]
                n163 = Unbundle(w260) -> (w256:string[])
                n164 = Match First String(2:w256, 3:w261) -> (0:w257:i32)  [unwired: 1 out]
                n165 = property on="Test Ring" class="Ring (strict)"("Value"=w257, "Strings []"=w256) -> ()  [unwired: 2 in, 2 out]
                n166 = property on="Test Ring" class="Ring (strict)"("Visible"=TRUE) -> ()  [unwired: 2 in, 2 out]
                n167 = property on="Test Slider" class="Slide (strict)"("Visible"=FALSE) -> ()  [unwired: 2 in, 2 out]
              }
              frame Default {
                n168 = property on="Test Ring" class="Ring (strict)"("Visible"=FALSE) -> ()  [unwired: 2 in, 2 out]
                n169 = property on="Test Slider" class="Slide (strict)"("Visible"=FALSE) -> ()  [unwired: 2 in, 2 out]
              }
              frame "Brightness  **", "Color Level  **", "Compression  **", "FPS  **", "Sharpness  **" {
                n170 = call <vilib>:"NT Read Number.vi"("Name"=w268) -> ("Numeric"=w267:dbl)  [unwired: 9 in, 1 out]
                n171 = local write "Test Slider"(w267) -> ()
                n172 = property on="Test Slider" class="Slide (strict)"("Visible"=TRUE, "Scale.Maximum"=100.0 ("Scale.Range:Maximum")) -> ()  [unwired: 2 in, 2 out]
                n173 = property on="Test Ring" class="Ring (strict)"("Visible"=FALSE) -> ()  [unwired: 2 in, 2 out]
              }
            }
          }
        }
        n174 = property on="Progress" class="Clust (strict)"("Visible"=FALSE) -> ()  [unwired: 2 in, 2 out]
      }
      event "Test Name": Mouse Enter {
        # "Populate the ring with the list of tests"
        n175 = event-data() -> ()  [unwired: 1 in, 1 out]
        n176 = call <vilib>:"NT Read String Array.vi"("Name"="TestMode/TestList") -> ("String Array"=w276:string[])  [unwired: 9 in, 1 out]
        n177 = Build Array (concatenate)("Select the test to run...", w276) -> (w275:string[])
        n178 = property on="Test Name" class="Ring (strict)"("Strings []"=w275) -> ()  [unwired: 2 in, 2 out]
      }
      event "Test Name": Value Change {
        w278 = FALSE ("Visible")
        # "Tell the robot the test name to run"
        n179 = event-data() -> ("NewVal"=w282:u16)  [unwired: 1 in]
        n180 = property on="Test Name" class="Ring (strict)"() -> ("Strings []"=w283:string[])  [unwired: 2 in, 2 out]
        n181 = local write "Progress"(T7 {"Test Progress"=0, "Test Progress Text"=""} ("Progress")) -> ()
        n182 = Index Array(array=w283, index=w282) -> (element=w281:string)
        n183 = call <vilib>:"NT Write String.vi"("String"=w281, "Name"="TestMode/TestName") -> ()  [unwired: 9 in, 1 out]
        n184 = property on="Progress" class="Clust (strict)"("Visible"=TRUE) -> ()  [unwired: 2 in, 2 out]
        n185 = property on="Motor" class="Clust (strict)"("Visible"=w278) -> ()  [unwired: 2 in, 2 out]
        n186 = property on="Test Slider" class="Slide (strict)"("Visible"=w278) -> ()  [unwired: 2 in, 2 out]
        n187 = property on="On/Off" class="Bool (strict)"("Visible"=w278) -> ()  [unwired: 2 in, 2 out]
        n188 = property on="Rev/Fwd" class="Clust (strict)"("Visible"=w278) -> ()  [unwired: 2 in, 2 out]
        n189 = property on="Test Ring" class="Ring (strict)"("Visible"=w278) -> ()  [unwired: 2 in, 2 out]
      }
      event "Listbox": Double Click {
        # "Shift clears all"
        # "Update symbols on the listbox"
        n190 = event-data() -> ("PlatMods.Shift"=w286:bool, "Row"=w288:i32)  [unwired: 1 in]
        n191 = case shown="True" w286 {
          tunnel: w288 -> [w292 _]
          tunnel: 1 -> [w291 _]
          frame False {
            n192 = property on="Listbox" class="LstBox (strict)"() -> ("Item Symbols"=w290:i32[])  [unwired: 2 in, 2 out]
            n193 = Replace Array Subset(array=w290, new element=w291, index=w292) -> (w289:i32[])
            n194 = property on="Listbox" class="LstBox (strict)"("Item Symbols"=w289) -> ()  [unwired: 2 in, 2 out]
          }
          frame True {
            w293 = 0 ("Top Row")
            n195 = property on="Listbox" class="LstBox (strict)"() -> ("Number of Rows"=w295:u32)  [unwired: 2 in, 2 out]
            n196 = Initialize Array(0, w295) -> (w294:i32[])
            n197 = property on="Listbox" class="LstBox (strict)"("Top Row"=w293, "Value"=w293, "Item Symbols"=w294) -> ()  [unwired: 2 in, 2 out]
          }
        }
      }
      event "Listbox": Key Down {
        # "Update symbols on the listbox\nLeft and right keys check and uncheck"
        n198 = event-data() -> ("VKey"=w299:T20)  [unwired: 1 in]
        n199 = case shown="\"Left\", \"Right\"" w299 {
          selector: w299 -> [w304 _]
          tunnel: eventvkey."Left" ("VKey") -> [w302 _]
          frame "Left", "Right" {
            n200 = Equal?(x=w302, y=w304) -> (x = y?=w303:bool)
            n201 = Select(t=0, s=w303, f=1) -> (s? t:f=w305:i32)
            n202 = property on="Listbox" class="LstBox (strict)"() -> ("Item Symbols"=w308:i32[])  [unwired: 2 in, 2 out]
            n203 = Replace Array Subset(array=w308, new element=w305, index="Listbox") -> (w307:i32[])
            n204 = property on="Listbox" class="LstBox (strict)"("Item Symbols"=w307) -> ()  [unwired: 2 in, 2 out]
          }
          frame Default {
          }
        }
      }
      event "DB Camera Config": Value Change {
        # "Show or hide the cluster of controls, store in ini file"
        n205 = event-data() -> ("NewVal"=w312:bool)  [unwired: 1 in]
        n206 = case shown="False" w312 {
          tunnel: w311 -> [w321 _]
          tunnel: [w314 w332] -> w310
          tunnel: w309 -> [w313 w332]
          frame False {
            w328 = "Camera"
            w331 = FALSE ("Visible")
            n207 = local read "Camera Settings"() -> (w320:T2)
            n208 = Index Array(array=w321) -> (element=w324:cluster{string[]})  [unwired: 1 in]
            n209 = Unbundle(w320) -> ("Frame Rate"=w319:i32, "Compression"=w318:i32, "Size"=w322:u16)
            n210 = Unbundle(w324) -> (w323:string[])
            n211 = Index Array(array=w323, index=w322) -> (element=w317:string)
            n212 = call-poly <vilib>:"Write Key.vi"("section"=w328, "value"=w317, "key"="Size", "refnum"=w313) -> ("refnum out"=w330:T18)  [unwired: 2 in, 5 out]
            n213 = call-poly <vilib>:"Write Key.vi"("section"=w328, "value"=w319, "key"="FrameRate", "refnum"=w330) -> ("refnum out"=w329:T18)  [unwired: 1 in, 6 out]
            n214 = property on="Camera Settings" class="Clust (strict)"("Visible"=w331) -> ()  [unwired: 2 in, 2 out]
            n215 = local write "DB Camera Config"(w331) -> ()
            n216 = call-poly <vilib>:"Write Key.vi"("section"=w328, "value"=w318, "key"="Compression", "refnum"=w329) -> ("refnum out"=w315:T18)  [unwired: 1 in, 6 out]
            n217 = call <vilib>:"Close Config Data.vi"("refnum"=w315) -> ("file path"=w316:path)  [unwired: 2 in, 8 out]
            n218 = call <vilib>:"Open Config Data.vi"("configuration file path"=w316) -> ("refnum"=w314:T18)  [unwired: 8 in, 2 out]
          }
          frame True {
            n219 = property on="Camera Settings" class="Clust (strict)"("Visible"=TRUE) -> ()  [unwired: 2 in, 2 out]
          }
        }
      }
      event "Camera Settings": Value Change {
        # "Update summary string when any elements of DB camera change"
        n220 = event-data() -> ("NewVal"=w345:T2)  [unwired: 1 in]
        n221 = Index Array(array=w341) -> (element=w340:cluster{string[]})  [unwired: 1 in]
        n222 = Unbundle(w345) -> ("Frame Rate"=w336:i32, "Compression"=w335:i32, "Size"=w338:u16)
        n223 = Unbundle(w340) -> (w339:string[])
        n224 = Index Array(array=w339, index=w338) -> (element=w337:string)
        n225 = Format Into String(format string="%s   %dfps   %d%%", w337, w336, w335) -> (resulting string=w342:string)  [unwired: 2 in, 1 out]
        n226 = Build Array(w342) -> (w343:string[])
        n227 = property on="DB Camera Config" class="Bool (strict)"("Strings [4]"=w343) -> ()  [unwired: 2 in, 2 out]
      }
      event "Motor.Enable": Value Change {
        # "When the test mode otor enable helper is set, update that\ntree row item's value"
        n228 = event-data() -> ("NewVal"=w351:bool)  [unwired: 1 in]
        n229 = Unbundle("Motor") -> ("Value"=w350:dbl)  [unwired: 1 out]
        n230 = Select(t=w350, s=w351, f=0.0) -> (s? t:f=w348:dbl)
        n231 = call <vilib>:"NT Write Number.vi"("Numeric"=w348, "Name"=w347) -> ()  [unwired: 9 in, 1 out]
      }
      event "Test Slider": Value Change {
        # "When the test mode slider helper is set, update that\ntree row item's value"
        n232 = event-data() -> ("NewVal"=w354:dbl)  [unwired: 1 in]
        n233 = call <vilib>:"NT Write Number.vi"("Numeric"=w354, "Name"=w355) -> ()  [unwired: 9 in, 1 out]
      }
      event "On/Off": Value Change {
        # "When the test mode on/off helper value is set, update that\ntree row item's value"
        n234 = event-data() -> ("NewVal"=w359:bool)  [unwired: 1 in]
        n235 = Boolean To (0,1)(Boolean=w359) -> (0, 1=w358:i16)
        n236 = call <vilib>:"NT Write Number.vi"("Numeric"=w358, "Name"=w357) -> ()  [unwired: 9 in, 1 out]
      }
      event "Rev/Fwd": Value Change {
        # "When the test mode helper value for relays is set, update that\ntree row item's value"
        n237 = event-data() -> ("NewVal.Forward"=w367:bool, "NewVal.Reverse"=w366:bool)  [unwired: 1 in]
        n238 = Boolean To (0,1)(Boolean=w367) -> (0, 1=w363:i16)
        n239 = Boolean To (0,1)(Boolean=w366) -> (0, 1=w365:i16)
        n240 = Negate(x=w365) -> (-x=w364:i16)
        n241 = Add(x=w363, y=w364) -> (x+y=w362:i16)
        n242 = call <vilib>:"NT Write Number.vi"("Numeric"=w362, "Name"=w361) -> ()  [unwired: 9 in, 1 out]
      }
      event "Test Ring": Value Change {
        # "When a test mode helper value is selected from the ring,\nset the tree item's variable to the string value"
        n243 = event-data() -> ("NewVal"=w371:u16)  [unwired: 1 in]
        n244 = property on="Test Ring" class="Ring (strict)"() -> ("Strings []"=w372:string[])  [unwired: 2 in, 2 out]
        n245 = Index Array(array=w372, index=w371) -> (element=w370:string)
        n246 = call <vilib>:"NT Write String.vi"("String"=w370, "Name"=w369) -> ()  [unwired: 9 in, 1 out]
      }
      event "Rec Mode": Value Change {
        # "Update globals for recording mode and path to read log from.\nClear when logging and let NetworkTables set path for vision to\nuse."
        n247 = event-data() -> ("NewVal"=w382:enum32{"Stop", "Record", "Playback"})  [unwired: 1 in]
        n248 = global write "WPI_DashboardLogging Global.vi" "Logging Filename"(path "") -> ()
        n249 = case shown="\"Playback\"" w382 {
          tunnel: w381 -> [_ w384 w392]
          tunnel: [_ _ w391] -> w378
          tunnel: [_ _ w390] -> _
          tunnel: w376 -> [_ _ w388]
          tunnel: cluster{i32, i32} {-250, 170} -> [_ _ w387]
          tunnel: [_ _ T21 {"Image Size"=TRUE, "Image Type"=TRUE, "Pixel Value"=TRUE, "ROI Information"=TRUE, "Zoom Factor"=FALSE} ("Image Information Shown:All Elements")] -> w374
          tunnel: [_ _ TRUE ("Zoom Factor")] -> w373
          frame Default {
          }
          frame "Stop", "Record" {
            # "Place Window too"
            n250 = invoke class="VI" method="FP.Close"(reference=w384) -> (reference out=w383:refnum<vi>)  [unwired: 2 in, 2 out]
            n251 = invoke class="VI" method="Abort VI"(reference=w383) -> ()  [unwired: 2 in, 3 out]
          }
          frame "Playback" {
            n252 = call "Open Playback Panel.vi"("Offset"=w387, "DB VI Ref"=w388, "Playback in"=w392) -> ("Playback out"=w389:refnum<vi>)  [unwired: 8 in]
            n253 = register-events(w389) -> (reference out=w391:refnum<event-registration>, error out=w390:errorcluster)  [unwired: 2 in]
          }
        }
        n254 = global write "WPI_DashboardLogging Global.vi" "Recording"(w382) -> ()
        n255 = property on="Camera Image" class="ImageControl"("Image Information Shown"=w374, "Image Information Visible"=w373) -> ()  [unwired: 2 in, 2 out]
        n256 = call <vilib>:"WPI_DashboardNT Log FieldName Cache.vi"("Operation"=enum16{"Lookup/Add", "Index", "Clear"}."Clear") -> ()  [unwired: 8 in, 3 out]
      }
      event Panel Close {
        w393 = enum32{"Stop", "Record", "Playback"}."Stop" ("Rec Mode")
        # "Playback window has been closed, abort"
        n257 = event-data() -> ()  [unwired: 1 in, 4 out]
        n258 = local write "Rec Mode"(w393) -> ()
        n259 = global write "WPI_DashboardLogging Global.vi" "Recording"(w393) -> ()
      }
      event Panel Close {
        # "Abort playback window and ourself"
        n260 = event-data() -> ()  [unwired: 1 in, 4 out]
        n261 = invoke class="VI" method="FP.Close"(reference=w398) -> (reference out=w397:refnum<vi>)  [unwired: 2 in, 2 out]
        n262 = invoke class="VI" method="Abort VI"(reference=w397) -> (error out=w396:errorcluster)  [unwired: 2 in, 2 out]
        n263 = invoke class="VI" method="Abort VI"(error in=w396) -> ()  [unwired: 2 in, 3 out]
      }
      event "Vision": Value Change {
        # "Enable/Disable Compression slider.\nHW USB is hard-coded into the camera"
        n264 = event-data() -> ("NewVal"=w404:u16)  [unwired: 1 in]
        n265 = Equal?(x=w404, y=u32 2 ("milliseconds to wait")) -> (x = y?=w402:bool)
        n266 = Select(t=T22."Disabled and Grayed Out" ("Disabled"), s=w402, f=T22."Enabled" ("Disabled")) -> (s? t:f=w399:T22)
        n267 = property on="Compression" class="Slide (strict)"("DisabledEnum"=w399) -> ()  [unwired: 2 in, 2 out]
      }
    }
  }
  n268 = while {
    tunnel: w38 -> [w407]
    i -> [w410]
    stop <- FALSE stop-if-true
    n269 = Wait (ms)(milliseconds to wait=u32 100) -> ()  [unwired: 1 out]
    n270 = case shown="\"Playback\"" "Rec Mode" {
      tunnel: w410 -> [_ _ w425]
      tunnel: [u32 2829099 ("Base Color") u32 11141120 ("Target Color") w414] -> w406
      frame "Stop", Default {
        # "Reset the color, extra updates don't cost much"
      }
      frame "Record" {
      }
      frame "Playback" {
        # "Playback"
        n271 = Quotient & Remainder(x=w425, y=u32 50 ("milliseconds to wait")) -> (x-y*floor(x/y)=w421:u32)  [unwired: 1 out]
        n272 = Divide(x=w421, y=u32 50 ("milliseconds to wait")) -> (x/y=w418:dbl)
        n273 = Multiply(x=6.283185307179586, y=w418) -> (x*y=w423:dbl)
        n274 = Sine(x=w423) -> (sin(x)=w422:dbl)
        n275 = Absolute Value(x=w422) -> (abs(x)=w415:dbl)
        n276 = call "Interpolate RGB Color.vi"("Proportion"=w415, "Target Color"=u32 30976, "Base Color"=u32 2829099) -> ("Result Color"=w414:u32)  [unwired: 8 in]
      }
    }
    n277 = property class="Pane"(reference=w407, "PaneColor"=w406) -> ()  [unwired: 1 in, 2 out]
  }
  n278 = TCP Create Listener(10:u16 1741 ("timeout ms (25000)")) -> (3:w1:refnum<k5>)  [unwired: 4 in, 2 out]
  n279 = while {
    tunnel: w1 -> [w427]
    stop <- FALSE stop-if-true
    n280 = TCP Wait On Listener(11:w427) -> (4:w426:refnum<k5>)  [unwired: 3 in, 4 out]
    n281 = local write "TCP"(w426) -> ()
  }
  n282 = property on="On/Off" class="Bool (strict)"("Visible"=w6) -> ()  [unwired: 2 in, 2 out]
  n283 = property on="Motor" class="Clust (strict)"("Visible"=w6) -> ()  [unwired: 2 in, 2 out]
  n284 = property on="Progress" class="Clust (strict)"("Visible"=w6) -> ()  [unwired: 2 in, 2 out]
  n285 = property on="Test Ring" class="Ring (strict)"("Visible"=w6) -> ()  [unwired: 2 in, 2 out]
  n286 = property on="Rev/Fwd" class="Clust (strict)"("Visible"=w6) -> ()  [unwired: 2 in, 2 out]
  n287 = property on="Camera Settings" class="Clust (strict)"("Visible"=w6) -> ()  [unwired: 2 in, 2 out]
  n288 = local write "DB Camera Config"(w6) -> ()
  n289 = global write "WPI_DashboardLogging Global.vi" "Recording"(w32) -> ()
  n290 = local write "Rec Mode"(w32) -> ()
